vi "clFileReader_writeStr.vi"(9 "offset":u32, 10 "ReadStr - IN Value":string, 11 "clFileReader.lvclass IN":refnum<class "clFileReader.lvclass">) -> (1 "new offset":u32, 3 "clFileReader.lvclass OUT":refnum<class "clFileReader.lvclass">)   [LabVIEW 2016, in "vi_lib.lvlib" / "clFileReader.lvclass"]
uses:
  clFileReader.lvclass
  clFileReader.lvclass/clFileReader.ctl
  clFile/clFile.lvclass
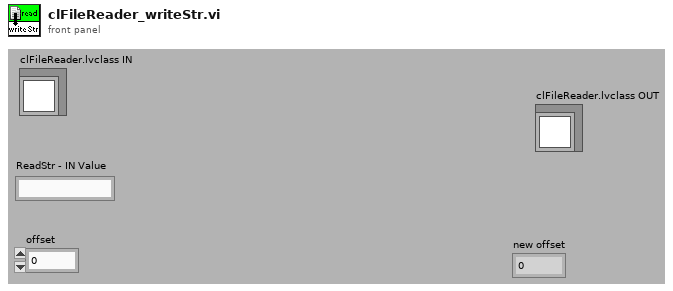
[diagram p1: front panel]
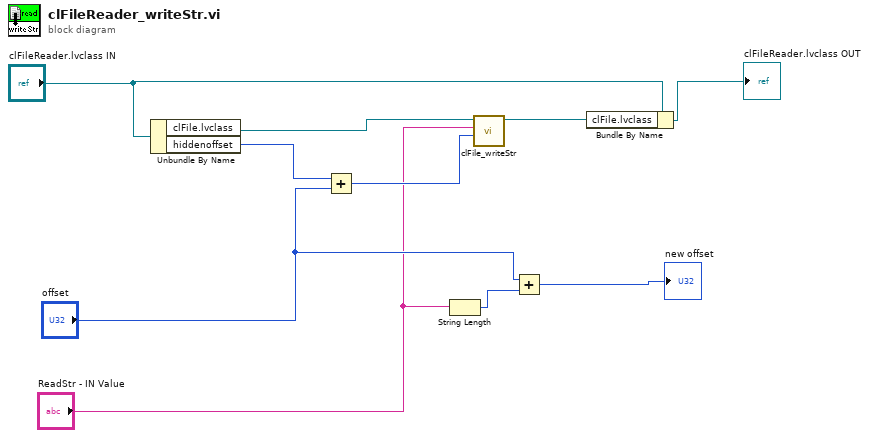
[diagram p0: block diagram]
diagram:
  n1 = Unbundle By Name("clFileReader.lvclass IN") -> ("clFile.lvclass"=w10:refnum<class "clFile.lvclass">, "hiddenoffset"=w9:u32)
  n2 = Add(x=w9, y="offset") -> (x+y=w8:u32)
  n3 = String Length(string="ReadStr - IN Value") -> (length=w5:i32)
  n4 = call "clFile_writeStr.vi"("offset (0)"=w8, "new substring"="ReadStr - IN Value", "clFile.lvclass"=w10) -> ("clFile.lvclass 2"=w2:refnum<class "clFile.lvclass">)  [unwired: 8 out]
  n5 = Add(x="offset", y=w5) -> (x+y=→"new offset":u32)
  n6 = Bundle By Name(cluster="clFileReader.lvclass IN", "clFile.lvclass"=w2) -> (→"clFileReader.lvclass OUT":refnum<class "clFileReader.lvclass">)
